vi "Hybrid Stop Read Server.vi"(1 "error in (no error)":errorcluster, 2 "vi reference":refnum<vi>) -> (0 "error out":errorcluster)   [LabVIEW 2025]
doc: "This is a simple example of a server which exports VIs to be called from another machine. You may run both the client.llb and server.llb on the same machine without modifying the access list. If you wish to run the client on another machine that is not in your domain you will have to list the name of the client in the Machine Access List. \n\nThe VIs listed in the Exported VI list are exported by the server.\n\nTo run this example start this VI First, then start the client.llb on all machines you want to try as clients. If you change either of the above lists, you must restart this VI for the changes to take effect.\n\nClick the \"Stop\" button to quit. This will turn off the server, terminating all client connections, and restore the previous access lists to their original values. \nAuthor: Scott Hannahs <sth@magnet.fsu.edu>\n\nThis software is licensed for use under the “MIT License\"\nCopyright (c) 2025 Scott Hannahs, sth@sth@magnet.sthnet.net\n\nPermission is hereby granted, free of charge, to any person obtaining a copy of this software and associated documentation files (the \"Software\"), to deal in the Software without restriction, including without limitation the rights to use, copy, modify, merge, publish, distribute, sublicense, and/or sell copies of the Software, and to permit persons to whom the Software is furnished to do so, subject to the following conditions: The above copyright notice and this permission notice shall be included in all copies or substantial portions of the Software.\n\nTHE SOFTWARE IS PROVIDED \"AS IS\", WITHOUT WARRANTY OF ANY KIND, EXPRESS OR IMPLIED, INCLUDING BUT NOT LIMITED TO THE WARRANTIES OF MERCHANTABILITY, FITNESS FOR A PARTICULAR PURPOSE AND NONINFRINGEMENT. IN NO EVENT SHALL THE AUTHORS OR COPYRIGHT HOLDERS BE LIABLE FOR ANY CLAIM, DAMAGES OR OTHER LIABILITY, WHETHER IN AN ACTION OF CONTRACT, TORT OR OTHERWISE, ARISING FROM, OUT OF OR IN CONNECTION WITH THE SOFTWARE OR THE USE OR OTHER DEALINGS IN THE SOFTWARE."
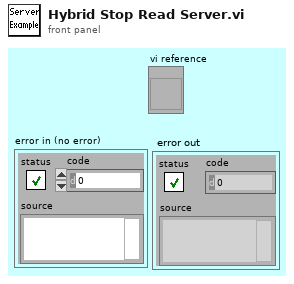
[diagram p1: front panel]
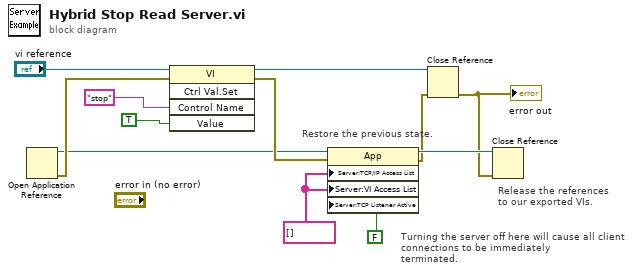
[diagram p0: block diagram]
diagram:
  w7 = string[] [] ("Server:TCP/IP Access List")
  # "Turning the server off here will cause all client connections to be immediately\nterminated."
  # "Release the references\nto our exported VIs."
  # "Restore the previous state."
  n1 = Open Application Reference() -> (0:w4:errorcluster, 3:w2:refnum<vi>)  [unwired: 4 in]
  n2 = invoke class="VI" method="Ctrl Val.Set"(reference="vi reference", error in=w4, "Control Name"="stop", "Value"=TRUE ("Server:TCP Listener Active")) -> (error out=w3:errorcluster)  [unwired: 1 in, 4 out]
  n3 = property class="App"(reference=w2, error in=w3, "Server:TCP/IP Access List"=w7, "Server:VI Access List"=w7, "Server:TCP Listener Active"=FALSE) -> (reference out=w11:refnum<vi>, error out=w10:errorcluster)
  n4 = Close Reference(reference="vi reference", error in (no error)=w10) -> (error out=w9:errorcluster)
  "error out" <- w9
  n5 = Close Reference(reference=w11, error in (no error)=w9) -> ()  [unwired: 1 out]
